vi "Get TDMs Contents.vi"   [LabVIEW 2012]
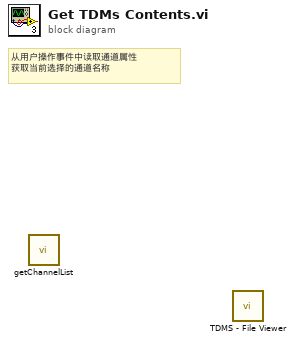
[diagram p0: block diagram]
diagram:
  # "从用户操作事件中读取通道属性\n获取当前选择的通道名称"
  n1 = call <vilib>:"getChannelList.vi"() -> ()  [unwired: 4 in, 4 out]
  n2 = call <vilib>:"TDMS - File Viewer.vi"() -> ()  [unwired: 6 in, 2 out]
